vi "Pre Launch Init.vi"(11 "SCADA in":refnum<class "SCADA.lvclass">) -> (0 "error out":errorcluster, 3 "SCADA out":refnum<class "SCADA.lvclass">)   [LabVIEW 2015, in "SCADA Core.lvlib" / "SCADA.lvclass"]
doc: "(<B>Filename</B>: Actor Framework.lvlib:Actor.lvclass:Pre Launch Init.vi)\n\nDefines behavior that occurs after the Launch Nested Actor method is invoked but before the actor's Actor Core method begins running.\n\nBy default, this method does nothing. A descendant class may override it to define behavior."
uses:
  SCADA.lvclass
  SCADA.lvclass/SCADA.ctl
  <vilib>/ActorFramework/Actor/Actor.lvclass
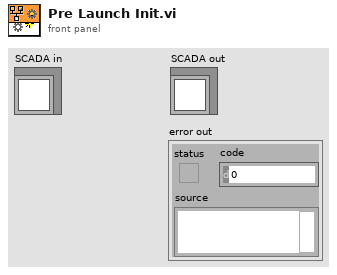
[diagram p1: front panel]
types:
  T1 = typedef "SCADA Core.lvlib/SCADA.lvclass/SCADA Core Notifiers.ctl" = cluster{"stop":refnum<notifier>, "SCADA stop":refnum<notifier>, "Logger stop":refnum<notifier>}
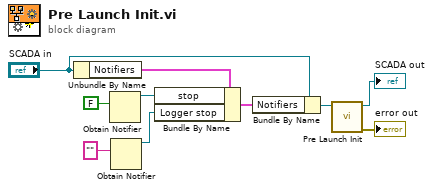
[diagram p0: block diagram]
diagram:
  n1 = Unbundle By Name("SCADA in") -> ("Notifiers"=w6:T1)
  n2 = Obtain Notifier(notification data type=FALSE) -> (notifier out=w4:refnum<notifier>)  [unwired: 3 in, 2 out]
  n3 = Obtain Notifier(notification data type="" ("f")) -> (notifier out=w1:refnum<notifier>)  [unwired: 3 in, 2 out]
  n4 = Bundle By Name(cluster=w6, "stop"=w4, "Logger stop"=w1) -> (w5:T1)
  n5 = Bundle By Name(cluster="SCADA in", "Notifiers"=w5) -> (w8:refnum<class "SCADA.lvclass">)
  n6 = call-parent "Pre Launch Init.vi"("Actor in"=w8) -> ("error out"=→"error out":errorcluster, "Actor out"=→"SCADA out":refnum<class "SCADA.lvclass">)  [unwired: 9 in]
